vi "channel data analyzer.vi"(11 "Channels":T1[](array[typedef])) -> ()   [LabVIEW 2012]
doc: "Analyze data portion of every received ARINC word in 1 channel. Ideally the data value should always increment by 1 if the simIO bitfile is used"
uses:
  RT/Typdefs/channel.ctl
  RT/Typdefs/received word.ctl
panel:
  out "dt":dbl(graph)
  out "value":u32(graph)
  in  "Ch index":i32
  # "should be always 1, otherwise a sample was missed"
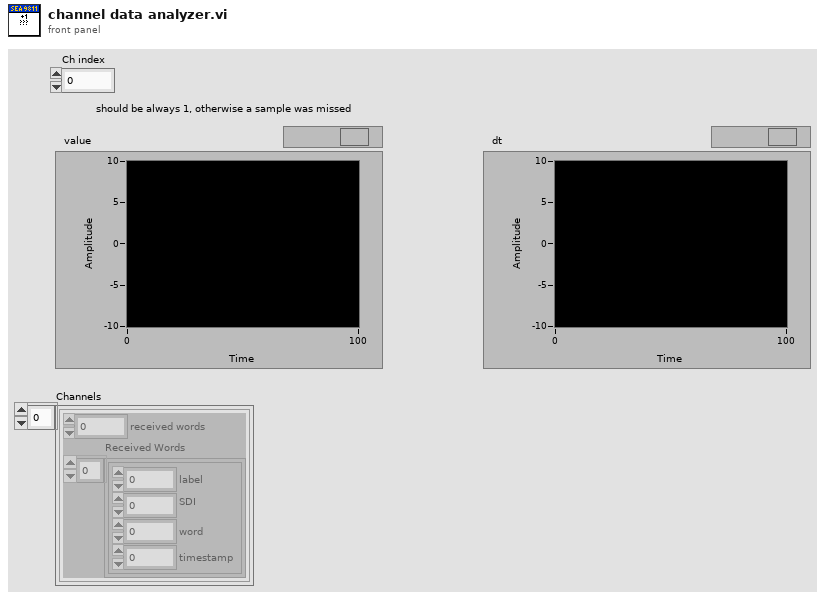
[diagram p1: front panel]
types:
  T1 = typedef "channel.ctl" = cluster{"received words":u32, "Received Words":T2[]}
  T2 = typedef "received word.ctl" = cluster{"label":u8, "SDI":u8, "word":u32, "timestamp":dbl}
  T3 = typedef "ARINC word cluster.ctl" = cluster{"ARINC word":T4, "Label":u8, "SDI":u8, "Data":u32, "Parity":bool, "timestamp (DBL)":dbl}
  T4 = typedef "ARINC word.ctl" = u32
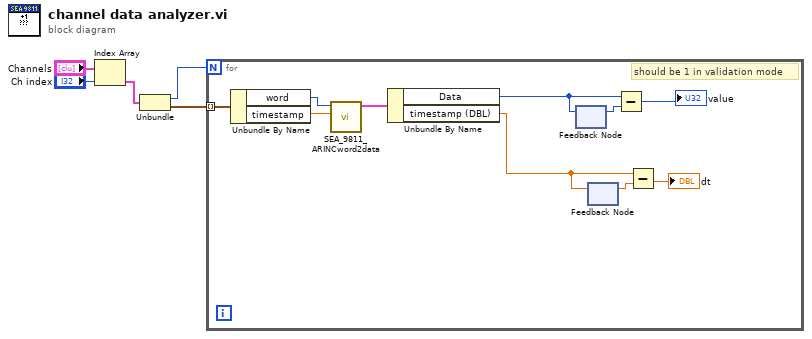
[diagram p0: block diagram]
diagram:
  n1 = Index Array(array="Channels", index="Ch index") -> (element=w5:T1)
  n2 = Unbundle(w5) -> ("received words"=w3:u32, "Received Words"=w2:T2[])
  n3 = for {
    N: w3 -> [_]
    tunnel: w2 -> [w15] mode=indexing
    # "should be 1 in validation mode"
    n4 = Unbundle By Name(w15) -> ("word"=w14:u32, "timestamp"=w13:dbl)
    n5 = call "SEA_9811_ARINCword2data.vi"("timestamp (DBL) in"=w13, "ARINC word in"=w14) -> ("ARINC word out"=w12:T3)  [unwired: 8 in, 1 out]
    n6 = Unbundle By Name(w12) -> ("Data"=w10:u32, "timestamp (DBL)"=w8:dbl)
    n7 = feedback-in #1(w10) -> ()
    n8 = feedback #1() -> (w11:u32)  [unwired: 1 in]
    n9 = feedback #2() -> (w9:dbl)  [unwired: 1 in]
    n10 = feedback-in #2(w8) -> ()
    n11 = Subtract(x=w10, y=w11) -> (x-y=→"value":u32)
    n12 = Subtract(x=w8, y=w9) -> (x-y=→"dt":dbl)
  }
